vi "linspace.vi"(9 "Samples":i32=5, 10 "Stop":dbl=1.0 format="%#_13g", 11 "Start":dbl=-1.0 format="%#_13g") -> (3 "Array":dbl[](array[numeric]))   [LabVIEW 2022 SP3]
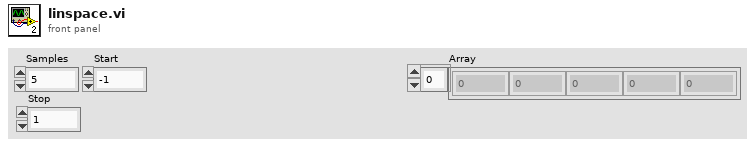
[diagram p1: front panel]
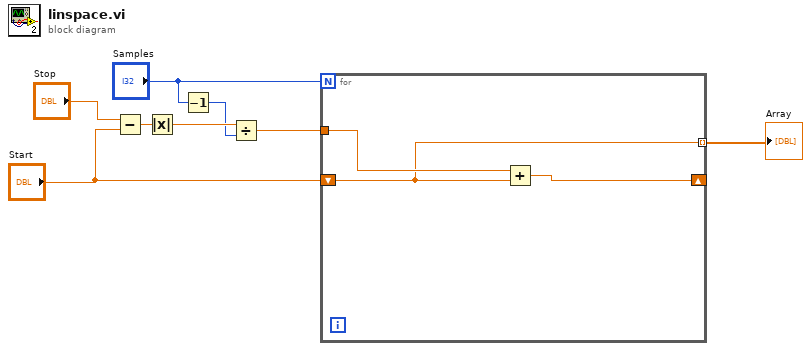
[diagram p0: block diagram]
diagram:
  n1 = Subtract(x="Stop", y="Start") -> (x-y=w8:dbl)
  n2 = Absolute Value(x=w8) -> (abs(x)=w6:dbl)
  n3 = Decrement(x="Samples") -> (x-1=w2:i32)
  n4 = Divide(x=w6, y=w2) -> (x/y=w5:dbl)
  n5 = for {
    N: "Samples" -> [_]
    tunnel: w5 -> [w11]
    shift-right: [w10] -> _
    shift-left: "Start" -> [w9]
    tunnel: [w9] -> w3 mode=indexing
    n6 = Add(x=w11, y=w9) -> (x+y=w10:dbl)
  }
  "Array" <- w3
